vi "control bank relay.vi"(8 "error in (no error)":errorcluster, 9 "Channel Data Reference":dbl, 10 "Connect Chn":T1, 11 "Refnum in":T2) -> (0 "error out":errorcluster)   [LabVIEW 2017, in "NI 272x Resistive Simulation Custom Device Engine.lvlib"]
uses:
  NI 272x Resistive Simulation Custom Device Engine.lvlib
  <instrlib>/ni272xReferenceVIs/ni272xReferenceVIs.llb/ni272x Reference.ctl
  Controls/Compiled Connect Channel.ctl
  <instrlib>/ni272xReferenceVIs/ni272xReferenceVIs.llb/ni272x Disconnect 2Bank.vi
  <instrlib>/ni272xReferenceVIs/ni272xReferenceVIs.llb/ni272x Connect 2Bank.vi
  NI 272x Resistive Simulation Custom Device Shared.lvlib
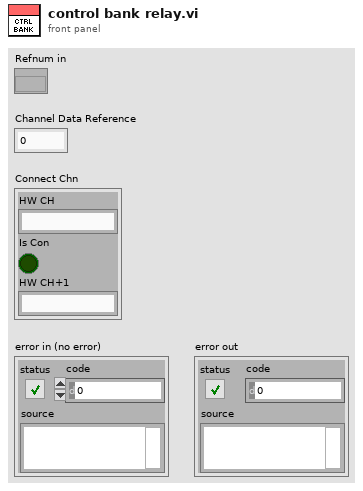
[diagram p1: front panel]
types:
  T1 = typedef "NI 272x Resistive Simulation Custom Device Shared.lvlib/Compiled Connect Channel.ctl" = cluster{"HW CH":string, "Is Con":bool, "HW CH+1":string}
  T2 = typedef "ni272x Reference.ctl" = refnum<k20>
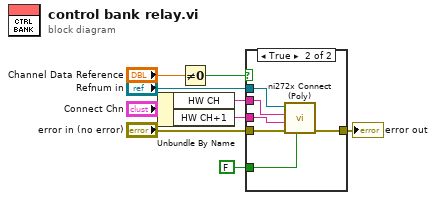
[diagram p0: block diagram]
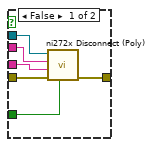
[diagram p2: hidden frame]
diagram:
  n1 = Unbundle By Name("Connect Chn") -> ("HW CH"=w3:string, "HW CH+1"=w4:string)
  n2 = Not Equal To 0?(x="Channel Data Reference") -> (x != 0?=w8:bool)
  n3 = case shown="True" w8 {
    tunnel: "Refnum in" -> [w15 w21]
    tunnel: w3 -> [w14 w20]
    tunnel: w4 -> [w13 w19]
    tunnel: "error in (no error)" -> [w12 w18]
    tunnel: [w11 w17] -> w6
    tunnel: FALSE ("wait for settling (T)") -> [w10 w16]
    frame False {
      n4 = call-poly <instrlib>:"ni272x Disconnect (Poly).vi"("wait for settling (T)"=w10, "error in (no error)"=w12, "resistor bank N+1"=w13, "resistor bank N"=w14, "instrument handle"=w15) -> ("error out"=w11:errorcluster)  [unwired: 5 in, 1 out]
    }
    frame True {
      n5 = call-poly <instrlib>:"ni272x Connect (Poly).vi"("wait for settling (T)"=w16, "error in (no error)"=w18, "resistor bank N+1"=w19, "resistor bank N"=w20, "instrument handle"=w21) -> ("error out"=w17:errorcluster)  [unwired: 5 in, 1 out]
    }
  }
  "error out" <- w6
